vi "delete assembly.vi"(8 "error in":errorcluster, 10 "instance ID":u32=100, 11 "EthernetIP configuration in":refnum<class "EthernetIP configuration.lvclass">) -> (0 "error out":errorcluster, 2 "invalidated channelsu":refnum<class "EthernetIP Channel.lvclass">[](array[class]), 3 "EthernetIP configuration out":refnum<class "EthernetIP configuration.lvclass">)   [LabVIEW 2013, in "EthernetIP configuration.lvclass"]
uses:
  EthernetIP configuration.lvclass
  channel/EthernetIP Channel.lvclass
  EthernetIP configuration.lvclass/EthernetIP configuration.ctl
  channel/EthernetIP Channel.lvclass/EthernetIP Channel.ctl
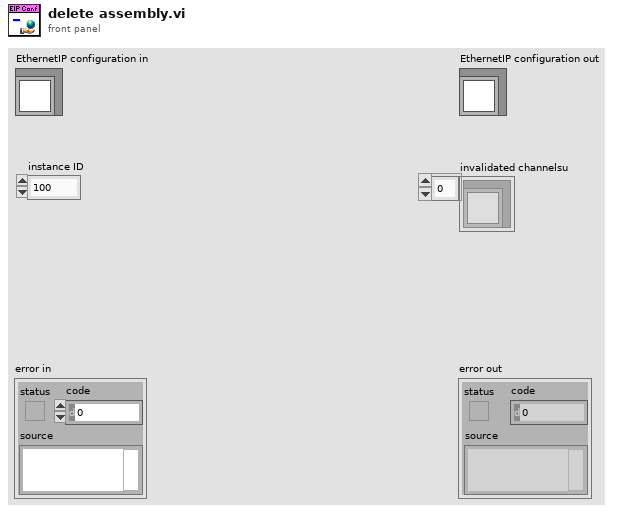
[diagram p1: front panel]
types:
  T1 = typedef "EthernetIP configuration.lvclass/assembly definition.ctl" = cluster{"name":string, "Instance ID":u32, "Type":T2, "Size (bytes)":u32}
  T2 = typedef "EthernetIP configuration.lvclass/assembly type.ctl" = enum32{"Producing", "Consuming"}
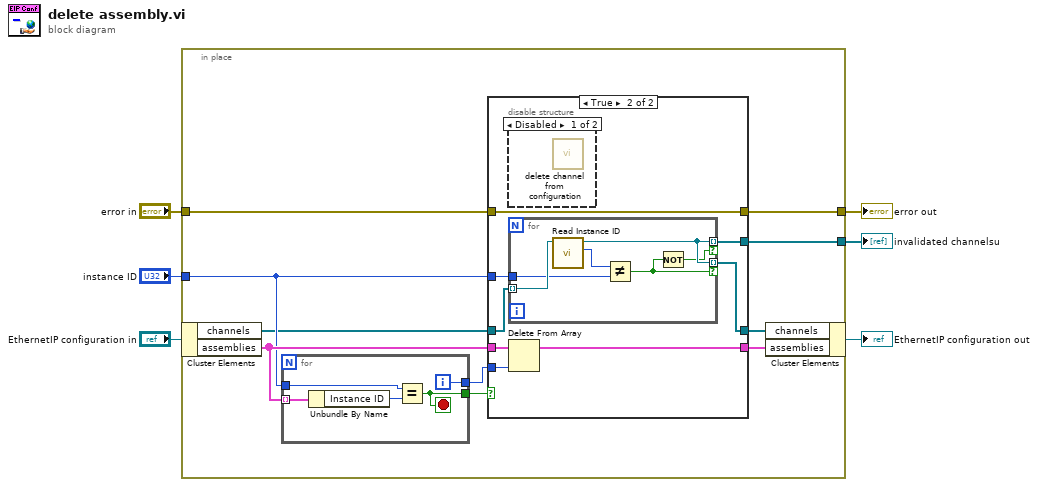
[diagram p0: block diagram]
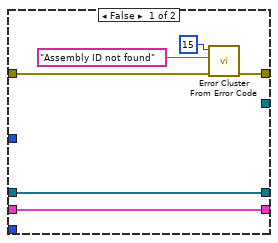
[diagram p2: hidden frame]
diagram:
  n1 = in-place {
    in-place-border: "instance ID" -> [w11]
    in-place-border: "error in" -> [w13]
    in-place-border: [w12] -> w2
    in-place-border: [w7] -> w1
    n2 = in-place-cluster #1("EthernetIP configuration in") -> ("channels"=w9:refnum<class "EthernetIP Channel.lvclass">[], "assemblies"=w14:T1[])
    n3 = for {
      tunnel: w14 -> [w41] mode=indexing
      tunnel: w11 -> [w39]
      tunnel: [w38] -> w16
      tunnel: [w37] -> w10
      i -> [w37]
      stop <- w38 stop-if-true
      n4 = Unbundle By Name(w41) -> ("Instance ID"=w40:u32)
      n5 = Equal?(x=w39, y=w40) -> (x = y?=w38:bool)
    }
    n6 = case shown="True" w16 {
      tunnel: [w22 w28] -> w15
      tunnel: w14 -> [w22 w29]
      tunnel: w13 -> [w19 w30]
      tunnel: [w18 w30] -> w12
      tunnel: w11 -> [_ w25]
      tunnel: w10 -> [_ w27]
      tunnel: w9 -> [w17 w26]
      tunnel: [w17 w24] -> w8
      tunnel: [_ w23] -> w7
      frame False {
        n7 = call <vilib>:"Error Cluster From Error Code.vi"("error in (no error)"=w19, "error message (\"\")"="Assembly ID not found" ("error message (\"\")"), "error code (0)"=15) -> ("error out"=w18:errorcluster)  [unwired: 6 in]
      }
      frame True {
        n8 = disable-structure shown="Disabled" {
          frame Disabled {
            n9 = call "delete channel from configuration.vi"() -> ()  [unwired: 10 in, 2 out]
          }
          frame Enabled {
          }
        }
        n10 = for {
          tunnel: w26 -> [w36] mode=indexing
          tunnel: w25 -> [w34]
          tunnel: [w33] -> w24 mode=indexing if=w32
          tunnel: [w33] -> w23 mode=indexing if=w31
          n11 = call "Read Instance ID.vi"("EthernetIP Channel in"=w36) -> ("Instance ID"=w35:u32, "EthernetIP Channel out"=w33:refnum<class "EthernetIP Channel.lvclass">)  [unwired: 8 in, 1 out]
          n12 = Not Equal?(x=w35, y=w34) -> (x != y?=w32:bool)
          n13 = Not(x=w32) -> (.not. x?=w31:bool)
        }
        n14 = Delete From Array(array=w29, index=w27) -> (array with subset deleted=w28:T1[])  [unwired: 1 in, 1 out]
      }
    }
    n15 = in-place-cluster #1("channels"=w8, "assemblies"=w15) -> (→"EthernetIP configuration out":refnum<class "EthernetIP configuration.lvclass">)
  }
  "error out" <- w2
  "invalidated channelsu" <- w1
